vi "SUMM.vi"() -> ()   [LabVIEW 2012]
panel:
  out "CF":bool
  out "S3":bool
  out "S2":bool
  out "S1":bool
  out "S0":bool
  in  "a3":bool
  in  "a2":bool
  in  "a1":bool
  in  "a0":bool
  in  "b3":bool
  in  "b2":bool
  in  "b 1":bool
  in  "b0":bool
  in  "op":bool
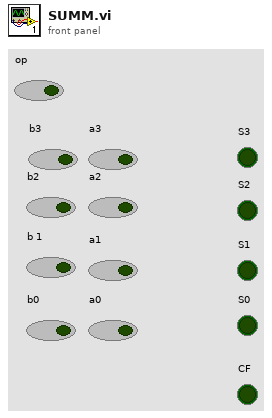
[diagram p1: front panel]
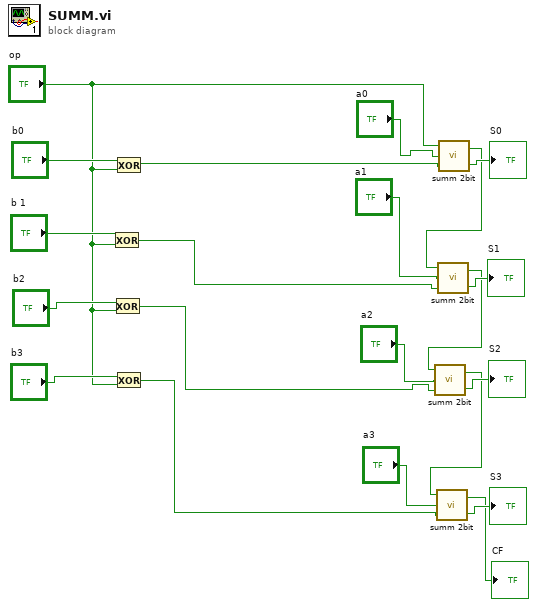
[diagram p0: block diagram]
diagram:
  n1 = Exclusive Or(1:"op", 2:"b 1") -> (0:w12:bool)
  n2 = Exclusive Or(1:"op", 2:"b2") -> (0:w4:bool)
  n3 = Exclusive Or(1:"op", 2:"b0") -> (0:w16:bool)
  n4 = Exclusive Or(1:"op", 2:"b3") -> (0:w2:bool)
  n5 = call "summ 2bit.vi"("b0"=w16, "a0"="a0", "C0"="op") -> ("S0"=→"S0":bool, "S1"=w14:bool)
  n6 = call "summ 2bit.vi"("b0"=w12, "a0"="a1", "C0"=w14) -> ("S0"=→"S1":bool, "S1"=w10:bool)
  n7 = call "summ 2bit.vi"("b0"=w4, "a0"="a2", "C0"=w10) -> ("S0"=→"S2":bool, "S1"=w7:bool)
  n8 = call "summ 2bit.vi"("b0"=w2, "a0"="a3", "C0"=w7) -> ("S0"=→"S3":bool, "S1"=→"CF":bool)
